vi "Begin.vi"(8 "error in":errorcluster) -> (0 "error out":errorcluster)   [LabVIEW 2016]
doc: "Called before other user functions, this VI can be used to open I/O refnums, load in file data, and do general program initialization. Notice that the <B>error out</B> terminal is simply used for data flow. Wiring it to other structures or subVIs ensures that this VI runs first."
uses:
  <vilib>/Rock Robotics/WPI/DriverStation/WPI_DriverStationRobotMode2.ctl
  <vilib>/Rock Robotics/WPI/Joystick/WPI_JoystickDeviceEnum.ctl
  <vilib>/Rock Robotics/SystemInterfaces/DIO/FPGA_DIOChannel.ctl
  <vilib>/Rock Robotics/WPI/Solenoid/WPI_SolenoidChannel.ctl
  <vilib>/Rock Robotics/SystemInterfaces/spilib/spi_bus.ctl
  <vilib>/Rock Robotics/WPI/SafetyOutput/WPI_SafetyOutputConfigMenu.ctl
  <vilib>/Rock Robotics/WPI/Encoder/WPI_EncoderType.ctl
  <vilib>/Rock Robotics/SystemInterfaces/DIO/FPGA_DIOPWMChannel.ctl
  <vilib>/Rock Robotics/SystemInterfaces/AI/FPGA_AIGyroChannel.ctl
  Robot Global Data.vi
  <vilib>/Rock Robotics/Network Tables/NT Write String Array.vi
  <vilib>/Rock Robotics/WPI/Counter/WPI_CounterDigitalInputToDigitalSource.vi
  <vilib>/Rock Robotics/WPI/Solenoid/WPI_SolenoidOpenDouble.vi
  <vilib>/Rock Robotics/WPI/MotorControl/WPI_MotorControlOpen SPARK.vi
  <vilib>/Rock Robotics/WPI/Gyro/WPI_GyroAnalogOpen.vi
  <vilib>/Rock Robotics/Network Tables/NT Read Number.vi
  <vilib>/Rock Robotics/WPI/Utilities/WPI_GetSetVariantRefNum.vi
  <vilib>/Rock Robotics/WPI/Solenoid/WPI_SolenoidOpenSingle.vi
  NavX/navX Library v2/navX Library v2.lvlib
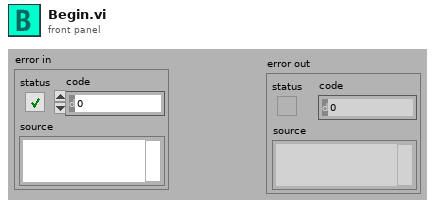
[diagram p1: front panel]
types:
  T1 = typedef "FPGA_AIGyroChannel.ctl" = enum8{"AI 0", "AI 1", "Invalid"}
  T2 = typedef "FPGA_DIOPWMChannel.ctl" = enum8{"PWM 0", "PWM 1", "PWM 2", "PWM 3", "PWM 4", "PWM 5", "PWM 6", "PWM 7", "PWM 8", "PWM 9", "PWM MXP 0", "PWM MXP 1", "PWM MXP 2", "PWM MXP 3", "PWM MXP 4", "PWM MXP 5", "PWM MXP 6", "PWM MXP 7", "PWM MXP 8", "PWM MXP 9", "Invalid"}
  T3 = typedef "FPGA_DIOChannel.ctl" = enum8{"DIO 0", "DIO 1", "DIO 2", "DIO 3", "DIO 4", "DIO 5", "DIO 6", "DIO 7", "DIO 8", "DIO 9", "DIO MXP 0", "DIO MXP 1", "DIO MXP 2", "DIO MXP 3", "DIO MXP 4", "DIO MXP 5", "DIO MXP 6", "DIO MXP 7", "DIO MXP 8", "DIO MXP 9", "DIO MXP 10", "DIO MXP 11", "DIO MXP 12", "DIO MXP 13", "DIO MXP 14", "DIO MXP 15", "SPI Port CS1", "SPI Port CS2", "SPI Port CS3", "SPI Port MISO", "SPI Port MOSI", "Invalid"}
  T4 = typedef "WPI_EncoderType.ctl" = enum16{"1x", "2x", "4x"}
  T5 = typedef "WPI_SafetyOutputConfigMenu.ctl" = enum16{"Enable", "Disable"}
  T6 = typedef "WPI_SolenoidChannel.ctl" = enum8{"Solenoid 0", "Solenoid 1", "Solenoid 2", "Solenoid 3", "Solenoid 4", "Solenoid 5", "Solenoid 6", "Solenoid 7", "Invalid"}
  T7 = typedef "WPI_JoystickDeviceEnum.ctl" = enum16{"USB 0", "USB 1", "USB 2", "USB 3", "USB 4", "USB 5"}
  T8 = typedef "spi_bus.ctl" = enum16{"SPI On-Board, CS0", "SPI On-Board, CS1", "SPI On-Board, CS2", "SPI On-Board, CS3", "SPI MXP", "Invalid"}
  T9 = typedef "WPI_DriverStationRobotMode2.ctl" = enum16{"Autonomous Disabled", "Autonomous Enabled", "Teleop Disabled", "Teleop Enabled", "Disconnected", "Finish", "Test Disabled", "Test Enabled", "Emergency Stopped"}
  T10 = typedef "WPI_CameraDevRef.ctl" = cluster{"Camera Address":string, "CameraStatus":errorcluster}
  T11 = typedef "WPI_GyroDevRef.ctl" = cluster{"DevStatus":errorcluster, "Analog Channel":T12, "Offset":dbl, "Gain (VoltsPerDegree/Second)":dbl, "Gyro Type":enum16{"Analog", "XRS450"}, "Handle":i32, "SPI Bus":T8, "Device Found":bool, "Sample Rate":dbl, "Calibrate On Open":bool}
  T12 = typedef "FPGA_AIChannel.ctl" = enum8{"AI 0", "AI 1", "AI 2", "AI 3", "AI MXP 0", "AI MXP 1", "AI MXP 2", "AI MXP 3", "Invalid"}
  T13 = typedef "WPI_JoystickDevRef.ctl" = cluster{"Device":T7}
  T14 = typedef "WPI_SolenoidDevRef.ctl" = cluster{"DevStatus":errorcluster, "Pneumatics Control Module":u8, "Forward Solenoid Channel":T6, "Reverse Solenoid Channel":T6}
  T15 = typedef "WPI_MotorControlDeviceRef.ctl" = cluster{"DeviceStatus":errorcluster, "Type":T16, "PWM":cluster{"PWM Channel":T2, "DeadBand":T17}, "CAN":cluster{"Device Number":u8, "SetOutput VI Ref":variant, "GetOutput VI Ref":variant, "Enable VI Ref":variant, "Disable VI Ref":variant, "Data":variant}, "Invert":bool}
  T16 = typedef "WPI_MotorControlType.ctl" = enum16{"PWM", "CAN"}
  T17 = typedef "WPI_PWMDeadband.ctl" = cluster{"Name":string, "maxPositivePwm":i32, "minPositivePwm":i32, "centerPwm":i32, "maxNegativePwm":i32, "minNegativePwm":i32, "angularRange":u16}
  T18 = typedef "WPI_DigitalInputDevRef.ctl" = cluster{"DevStatus":errorcluster, "DIO Channel":T3}
  T19 = typedef "FPGA_CounterEncoderSourceConvertionLVSourceType.ctl" = cluster{"DevStatus":errorcluster, "AnalogTriggerMode?":bool, "DigitalMode":cluster{"DIO Channel":T20}, "AnalogTriggerMode":cluster{"AnalogTriggerIndex":T21, "OutputType":T22}}
  T20 = typedef "FPGA_DIODigitalSourceChannel.ctl" = enum8{"DIO 0", "DIO 1", "DIO 2", "DIO 3", "DIO 4", "DIO 5", "DIO 6", "DIO 7", "DIO 8", "DIO 9", "DIO MXP 0", "DIO MXP 1", "DIO MXP 2", "DIO MXP 3", "DIO MXP 4", "DIO MXP 5", "DIO MXP 6", "DIO MXP 7", "DIO MXP 8", "DIO MXP 9", "DIO MXP 10", "DIO MXP 11", "DIO MXP 12", "DIO MXP 13", "DIO MXP 14", "DIO MXP 15", "Disabled"}
  T21 = typedef "FPGA_AnalogTriggerIndex.ctl" = enum8{"Trig 0", "Trig 1", "Trig 2", "Trig 3", "Trig 4", "Trig 5", "Trig 6", "Trig 7", "Invalid"}
  T22 = typedef "FPGA_AnalogTriggerOutType.ctl" = enum16{"InWindow", "TriggerState", "Rising", "Falling"}
  T23 = typedef "WPI_EncoderDevRef.ctl" = cluster{"DevStatus":errorcluster, "EncoderIndex":T24, "CounterIndex":T25, "DistancePerCount":dbl, "Decoding Type":T4}
  T24 = typedef "FPGA_EncoderIdx.ctl" = enum8{"Enc 0", "Enc 1", "Enc 2", "Enc 3", "Enc 4", "Enc 5", "Enc 6", "Enc 7", "Invalid"}
  T25 = typedef "FPGA_CounterCtrSystemIndex.ctl" = enum8{"Ctr 0", "Ctr 1", "Ctr 2", "Ctr 3", "Ctr 4", "Ctr 5", "Ctr 6", "Ctr 7", "Invalid"}
  T26 = typedef "navX Library v2.lvlib/Z900_navX_DeviceTypeDef.ctl" = cluster{"Interface":cluster{"Protocol":T27, "Update Rate (4Hz-60Hz)":u8, "navX Open TypeDef":variant}, "Notify Packet":refnum<notifier>, "Loop VI Refnum":refnum<vi>, "Ready to Close Occurrence Refnum":refnum<k4>}
  T27 = typedef "navX Library v2.lvlib/Z900_navX_ProtocolTypeDef.ctl" = enum16{"SERIAL", "I2C", "SPI"}
  T28 = cluster{"Yaw":dbl, "Roll":dbl, "Pitch":dbl, "Heading":dbl, "Fused Heading":dbl}
  T29 = typedef "WPI_CompressorDevRef.ctl" = cluster{"DevStatus":errorcluster, "Pneumatics Control Module":u8}
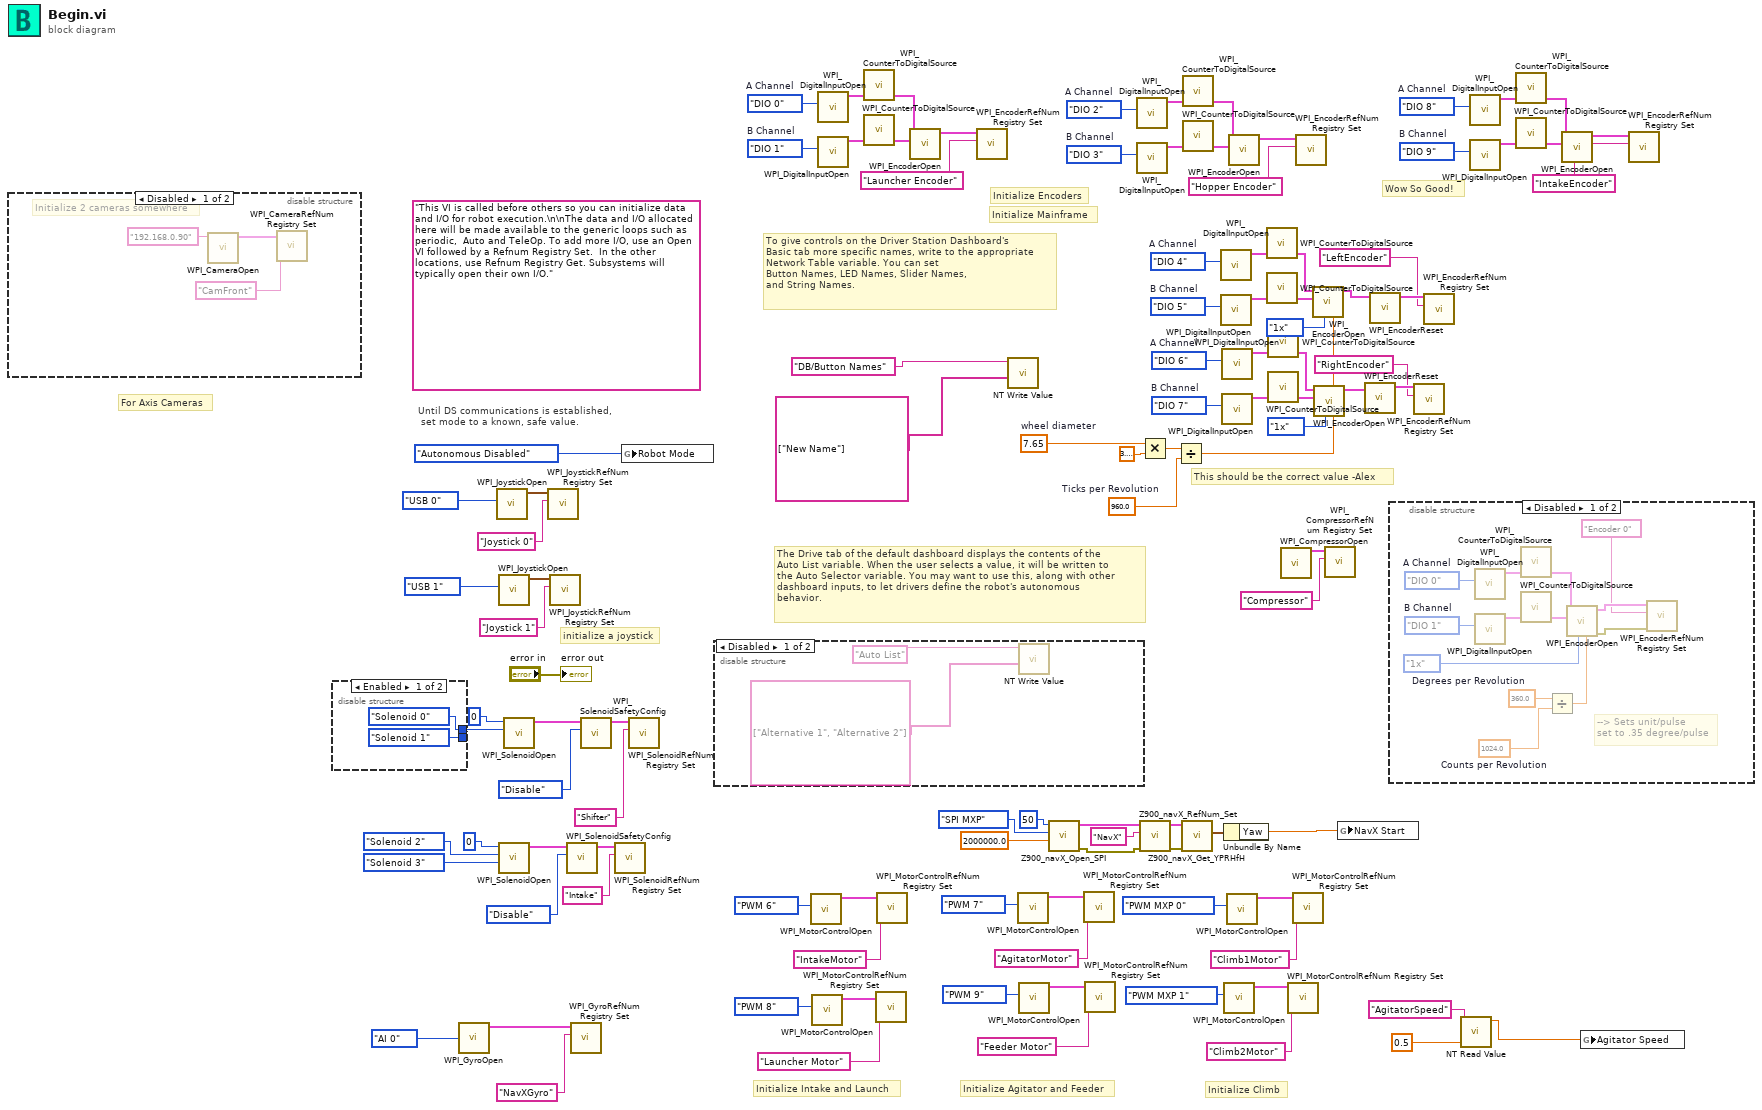
[diagram p0: block diagram]
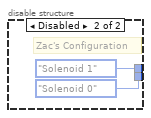
[diagram p4: hidden frame]
diagram:
  w25 = FPGA_DIOChannel."DIO 9"  # B Channel
  w26 = FPGA_DIOChannel."DIO 8"  # A Channel
  w41 = FPGA_DIOChannel."DIO 3"  # B Channel
  w42 = FPGA_DIOChannel."DIO 2"  # A Channel
  w33 = FPGA_DIOChannel."DIO 1"  # B Channel
  w34 = FPGA_DIOChannel."DIO 0"  # A Channel
  w52 = 960.0  # Ticks per Revolution
  w50 = 7.65  # wheel diameter
  w70 = FPGA_DIOChannel."DIO 5"  # B Channel
  w73 = FPGA_DIOChannel."DIO 4"  # A Channel
  w94 = FPGA_DIOChannel."DIO 7"  # B Channel
  w97 = FPGA_DIOChannel."DIO 6"  # A Channel
  (unwired) "This VI is called before others so you can initialize data and I/O for robot execution.\n\nThe data and I/O allocated here will be made available to the generic loops such as periodic,  Auto and TeleOp. To add more I/O, use an Open VI followed by a Refnum Registry Set.  In the other locations, use Refnum Registry Get. Subsystems will typically open their own I/O."
  # "Initialize Climb"
  # "Initialize Agitator and Feeder"
  # "Initialize Intake and Launch"
  # "For Axis Cameras"
  # "Wow So Good!"
  # "Initialize Mainframe"
  # "Initialize Encoders"
  # "This should be the correct value -Alex"
  # "The Drive tab of the default dashboard displays the contents of the\nAuto List variable. When the user selects a value, it will be written to\nthe Auto Selector variable. You may want to use this, along with other\ndashboard inputs, to let drivers define the robot's autonomous\nbehavior."
  # "To give controls on the Driver Station Dashboard's\nBasic tab more specific names, write to the appropriate\nNetwork Table variable. You can set\nButton Names, LED Names, Slider Names,\nand String Names."
  # "initialize a joystick"
  # "Until DS communications is established,\n set mode to a known, safe value."
  n1 = disable-structure shown="Disabled" {
    frame Disabled {
      # "Initialize 2 cameras somewhere"
      n2 = call <vilib>:"WPI_CameraOpen.vi"("Camera Address"="192.168.0.90") -> ("CameraDevRef"=w111:T10)  [unwired: 9 in, 1 out]
      n3 = call <vilib>:"WPI_CameraRefNum Registry Set.vi"("refnum name"="CamFront", "CameraDevRef"=w111) -> ()  [unwired: 8 in, 2 out]
    }
    frame Enabled {
    }
  }
  n4 = disable-structure shown="Enabled" {
    disable-tunnel: [WPI_SolenoidChannel."Solenoid 0" ("Solenoid Channel") WPI_SolenoidChannel."Solenoid 1" ("Solenoid Channel")] -> w79
    disable-tunnel: [WPI_SolenoidChannel."Solenoid 1" ("Reverse Solenoid Channel") WPI_SolenoidChannel."Solenoid 0" ("Reverse Solenoid Channel")] -> _
    frame Enabled {
    }
    frame Disabled {
      # "Zac's Configuration"
    }
  }
  n5 = call-poly <vilib>:"WPI_GyroOpen.vi"("Analog Channel"=FPGA_AIGyroChannel."AI 0") -> ("GyroDevRef"=w5:T11)  [unwired: 8 in, 2 out]
  n6 = call <vilib>:"WPI_JoystickOpen.vi"("JoystickDevice"=WPI_JoystickDeviceEnum."USB 0") -> ("JoystickDevRef"=w106:T13)  [unwired: 10 in]
  n7 = call <vilib>:"WPI_JoystickOpen.vi"("JoystickDevice"=WPI_JoystickDeviceEnum."USB 1") -> ("JoystickDevRef"=w68:T13)  [unwired: 10 in]
  n8 = call-poly <vilib>:"WPI_SolenoidOpen.vi"("Reverse Solenoid Channel"=WPI_SolenoidChannel."Solenoid 3", "Forward Solenoid Channel"=WPI_SolenoidChannel."Solenoid 2" ("Solenoid Channel"), "Pneumatics Control Module (0)"=u8 0) -> ("SolenoidDevRef"=w92:T14)  [unwired: 7 in, 1 out]
  n9 = call-poly <vilib>:"WPI_SolenoidOpen.vi"("Solenoid Channel"=w79, "Pneumatics Control Module (0)"=u8 0) -> ("SolenoidDevRef"=w62:T14)  [unwired: 8 in, 1 out]
  n10 = call <vilib>:"WPI_JoystickRefNum Registry Set.vi"("refnum name"="Joystick 0", "JoystickDevRef"=w106) -> ()  [unwired: 8 in, 2 out]
  n11 = call <vilib>:"WPI_JoystickRefNum Registry Set.vi"("refnum name"="Joystick 1", "JoystickDevRef"=w68) -> ()  [unwired: 8 in, 2 out]
  n12 = call <vilib>:"WPI_SolenoidSafetyConfig.vi"("mode"=WPI_SafetyOutputConfigMenu."Disable", "SolenoidDevRef"=w92) -> ("SolenoidDevRef"=w59:T14)  [unwired: 8 in, 1 out]
  n13 = call <vilib>:"WPI_GyroRefNum Registry Set.vi"("refnum name"="NavXGyro", "GyroDevRef"=w5) -> ()  [unwired: 8 in, 2 out]
  n14 = call <vilib>:"WPI_SolenoidSafetyConfig.vi"("mode"=WPI_SafetyOutputConfigMenu."Disable", "SolenoidDevRef"=w62) -> ("SolenoidDevRef"=w61:T14)  [unwired: 8 in, 1 out]
  n15 = call <vilib>:"WPI_SolenoidRefNum Registry Set.vi"("refnum name"="Intake", "SolenoidDevRef"=w59) -> ()  [unwired: 8 in, 2 out]
  n16 = global write "Robot Global Data.vi" "Robot Mode"(WPI_DriverStationRobotMode2."Autonomous Disabled" ("Robot Mode")) -> ()
  n17 = call <vilib>:"WPI_SolenoidRefNum Registry Set.vi"("refnum name"="Shifter", "SolenoidDevRef"=w61) -> ()  [unwired: 8 in, 2 out]
  n18 = disable-structure shown="Disabled" {
    frame Disabled {
      n19 = call-poly <vilib>:"NT Write Value.vi"("String Array"=string[] ["Alternative 1", "Alternative 2"], "Name"="Auto List") -> ()  [unwired: 9 in, 1 out]
    }
    frame Enabled {
    }
  }
  n20 = call-poly <vilib>:"WPI_MotorControlOpen.vi"("PWM Channel"=FPGA_DIOPWMChannel."PWM 6") -> ("MotorControlDeviceRef"=w11:T15)  [unwired: 9 in, 1 out]
  n21 = call-poly <vilib>:"WPI_MotorControlOpen.vi"("PWM Channel"=FPGA_DIOPWMChannel."PWM 8") -> ("MotorControlDeviceRef"=w8:T15)  [unwired: 9 in, 1 out]
  n22 = call <vilib>:"WPI_DigitalInputOpen.vi"("DIO Channel"=w34) -> ("DigitalInputDevRef"=w37:T18)  [unwired: 1 in, 9 out]
  n23 = call <vilib>:"WPI_DigitalInputOpen.vi"("DIO Channel"=w33) -> ("DigitalInputDevRef"=w36:T18)  [unwired: 1 in, 9 out]
  n24 = call-poly <vilib>:"WPI_CounterToDigitalSource.vi"("DigitalInputDevRef"=w37) -> ("Digital Source"=w38:T19)  [unwired: 6 out]
  n25 = call-poly <vilib>:"WPI_CounterToDigitalSource.vi"("DigitalInputDevRef"=w36) -> ("Digital Source"=w35:T19)  [unwired: 6 out]
  n26 = call <vilib>:"WPI_MotorControlRefNum Registry Set.vi"("refnum name"="Launcher Motor", "MotorControlDevRef"=w8) -> ()  [unwired: 8 in, 2 out]
  n27 = call <vilib>:"WPI_MotorControlRefNum Registry Set.vi"("refnum name"="IntakeMotor", "MotorControlDevRef"=w11) -> ()  [unwired: 8 in, 2 out]
  n28 = call <vilib>:"WPI_EncoderOpen.vi"("BSource"=w35, "ASource"=w38) -> ("EncoderDevRef"=w39:T23)  [unwired: 6 in, 3 out]
  n29 = call <vilib>:"WPI_EncoderRefNum Registry Set.vi"("refnum name"="Launcher Encoder", "EncoderDevRef"=w39) -> ()  [unwired: 8 in, 2 out]
  n30 = call-poly <vilib>:"NT Write Value.vi"("String Array"=string[] ["New Name"], "Name"="DB/Button Names") -> ()  [unwired: 9 in, 1 out]
  n31 = call-poly <vilib>:"WPI_MotorControlOpen.vi"("PWM Channel"=FPGA_DIOPWMChannel."PWM 7") -> ("MotorControlDeviceRef"=w14:T15)  [unwired: 9 in, 1 out]
  n32 = call-poly <vilib>:"WPI_MotorControlOpen.vi"("PWM Channel"=FPGA_DIOPWMChannel."PWM 9") -> ("MotorControlDeviceRef"=w16:T15)  [unwired: 9 in, 1 out]
  n33 = call "Z900_navX_Open_SPI.vi"("Clock Rate (Hz)"=2000000.0, "SPI Bus"=spi_bus."SPI MXP", "Update Rate (4Hz-60Hz)"=u8 50) -> ("error out"=w57:errorcluster, "navX Device"=w85:T26)  [unwired: 7 in]
  n34 = call <vilib>:"WPI_MotorControlRefNum Registry Set.vi"("refnum name"="AgitatorMotor", "MotorControlDevRef"=w14) -> ()  [unwired: 8 in, 2 out]
  n35 = call <vilib>:"WPI_MotorControlRefNum Registry Set.vi"("refnum name"="Feeder Motor", "MotorControlDevRef"=w16) -> ()  [unwired: 8 in, 2 out]
  n36 = call <vilib>:"WPI_DigitalInputOpen.vi"("DIO Channel"=w42) -> ("DigitalInputDevRef"=w45:T18)  [unwired: 1 in, 9 out]
  n37 = call <vilib>:"WPI_DigitalInputOpen.vi"("DIO Channel"=w41) -> ("DigitalInputDevRef"=w44:T18)  [unwired: 1 in, 9 out]
  n38 = Multiply(x=w50, y=3.141592653589793) -> (x*y=w53:dbl)
  n39 = call "Z900_navX_RefNum_Set.vi"("error in (no error)"=w57, "refnum name"="NavX", "navX Device"=w85) -> ("error out"=w56:errorcluster, "navX Device"=w86:T26)  [unwired: 7 in]
  n40 = Divide(x=w53, y=w52) -> (x/y=w49:dbl)
  n41 = call "Z900_navX_Get_YPRHfH.vi"("error in (no error)"=w56, "navX Device"=w86) -> ("YRPHfH"=w87:T28)  [unwired: 6 in, 3 out]
  n42 = call-poly <vilib>:"WPI_CounterToDigitalSource.vi"("DigitalInputDevRef"=w45) -> ("Digital Source"=w46:T19)  [unwired: 6 out]
  n43 = call-poly <vilib>:"WPI_CounterToDigitalSource.vi"("DigitalInputDevRef"=w44) -> ("Digital Source"=w43:T19)  [unwired: 6 out]
  n44 = call <vilib>:"WPI_DigitalInputOpen.vi"("DIO Channel"=w73) -> ("DigitalInputDevRef"=w74:T18)  [unwired: 1 in, 9 out]
  n45 = call <vilib>:"WPI_DigitalInputOpen.vi"("DIO Channel"=w70) -> ("DigitalInputDevRef"=w71:T18)  [unwired: 1 in, 9 out]
  n46 = call <vilib>:"WPI_DigitalInputOpen.vi"("DIO Channel"=w97) -> ("DigitalInputDevRef"=w98:T18)  [unwired: 1 in, 9 out]
  n47 = call <vilib>:"WPI_DigitalInputOpen.vi"("DIO Channel"=w94) -> ("DigitalInputDevRef"=w95:T18)  [unwired: 1 in, 9 out]
  n48 = Unbundle By Name(w87) -> ("Yaw"=w88:dbl)
  n49 = call-poly <vilib>:"WPI_MotorControlOpen.vi"("PWM Channel"=FPGA_DIOPWMChannel."PWM MXP 1") -> ("MotorControlDeviceRef"=w20:T15)  [unwired: 9 in, 1 out]
  n50 = call-poly <vilib>:"WPI_MotorControlOpen.vi"("PWM Channel"=FPGA_DIOPWMChannel."PWM MXP 0") -> ("MotorControlDeviceRef"=w22:T15)  [unwired: 9 in, 1 out]
  n51 = call <vilib>:"WPI_EncoderOpen.vi"("BSource"=w43, "ASource"=w46) -> ("EncoderDevRef"=w47:T23)  [unwired: 6 in, 3 out]
  n52 = call-poly <vilib>:"WPI_CounterToDigitalSource.vi"("DigitalInputDevRef"=w74) -> ("Digital Source"=w75:T19)  [unwired: 6 out]
  n53 = call-poly <vilib>:"WPI_CounterToDigitalSource.vi"("DigitalInputDevRef"=w71) -> ("Digital Source"=w72:T19)  [unwired: 6 out]
  n54 = call-poly <vilib>:"WPI_CounterToDigitalSource.vi"("DigitalInputDevRef"=w98) -> ("Digital Source"=w99:T19)  [unwired: 6 out]
  n55 = call-poly <vilib>:"WPI_CounterToDigitalSource.vi"("DigitalInputDevRef"=w95) -> ("Digital Source"=w96:T19)  [unwired: 6 out]
  n56 = call <vilib>:"WPI_CompressorOpen.vi"() -> ("CompressorDevRef"=w64:T29)  [unwired: 14 in, 1 out]
  n57 = call <vilib>:"WPI_MotorControlRefNum Registry Set.vi"("refnum name"="Climb2Motor", "MotorControlDevRef"=w20) -> ()  [unwired: 8 in, 2 out]
  n58 = call <vilib>:"WPI_MotorControlRefNum Registry Set.vi"("refnum name"="Climb1Motor", "MotorControlDevRef"=w22) -> ()  [unwired: 8 in, 2 out]
  n59 = call <vilib>:"WPI_EncoderRefNum Registry Set.vi"("refnum name"="Hopper Encoder", "EncoderDevRef"=w47) -> ()  [unwired: 8 in, 2 out]
  n60 = call <vilib>:"WPI_EncoderOpen.vi"("DistancePerCount"=w49, "Decoding Type"=WPI_EncoderType."1x", "BSource"=w72, "ASource"=w75) -> ("EncoderDevRef"=w76:T23)  [unwired: 4 in, 3 out]
  n61 = call <vilib>:"WPI_EncoderOpen.vi"("DistancePerCount"=w49, "Decoding Type"=WPI_EncoderType."1x", "BSource"=w96, "ASource"=w99) -> ("EncoderDevRef"=w100:T23)  [unwired: 4 in, 3 out]
  n62 = call <vilib>:"WPI_CompressorRefNum Registry Set.vi"("refnum name"="Compressor", "CompressorDevRef"=w64) -> ()  [unwired: 8 in, 2 out]
  n63 = global write "Robot Global Data.vi" "NavX Start"(w88) -> ()
  n64 = call <vilib>:"WPI_EncoderReset.vi"("EncoderDevRef"=w100) -> ("EncoderDevRef"=w101:T23)  [unwired: 9 in, 1 out]
  n65 = call <vilib>:"WPI_EncoderReset.vi"("EncoderDevRef"=w76) -> ("EncoderDevRef"=w77:T23)  [unwired: 9 in, 1 out]
  n66 = disable-structure shown="Disabled" {
    frame Disabled {
      w118 = 360.0  # Degrees per Revolution
      w121 = 1024.0  # Counts per Revolution
      w130 = FPGA_DIOChannel."DIO 1"  # B Channel
      w129 = FPGA_DIOChannel."DIO 0"  # A Channel
      # "--> Sets unit/pulse\nset to .35 degree/pulse"
      n67 = call <vilib>:"WPI_DigitalInputOpen.vi"("DIO Channel"=w129) -> ("DigitalInputDevRef"=w126:T18)  [unwired: 1 in, 9 out]
      n68 = call <vilib>:"WPI_DigitalInputOpen.vi"("DIO Channel"=w130) -> ("DigitalInputDevRef"=w127:T18)  [unwired: 1 in, 9 out]
      n69 = call-poly <vilib>:"WPI_CounterToDigitalSource.vi"("DigitalInputDevRef"=w126) -> ("Digital Source"=w125:T19)  [unwired: 6 out]
      n70 = call-poly <vilib>:"WPI_CounterToDigitalSource.vi"("DigitalInputDevRef"=w127) -> ("Digital Source"=w128:T19)  [unwired: 6 out]
      n71 = Divide(x=w118, y=w121) -> (x/y=w120:dbl)
      n72 = call <vilib>:"WPI_EncoderOpen.vi"("DistancePerCount"=w120, "Decoding Type"=WPI_EncoderType."1x", "BSource"=w128, "ASource"=w125) -> ("error out"=w123:errorcluster, "EncoderDevRef"=w124:T23)  [unwired: 4 in, 2 out]
      n73 = call <vilib>:"WPI_EncoderRefNum Registry Set.vi"("error in (no error)"=w123, "refnum name"="Encoder 0", "EncoderDevRef"=w124) -> ()  [unwired: 7 in, 2 out]
    }
    frame Enabled {
    }
  }
  n74 = call <vilib>:"WPI_EncoderRefNum Registry Set.vi"("refnum name"="RightEncoder", "EncoderDevRef"=w101) -> ()  [unwired: 8 in, 2 out]
  n75 = call <vilib>:"WPI_EncoderRefNum Registry Set.vi"("refnum name"="LeftEncoder", "EncoderDevRef"=w77) -> ()  [unwired: 8 in, 2 out]
  n76 = call-poly <vilib>:"NT Read Value.vi"("Default Value"=0.5, "Name"="AgitatorSpeed") -> ("Numeric"=w1:dbl)  [unwired: 8 in, 1 out]
  n77 = call <vilib>:"WPI_DigitalInputOpen.vi"("DIO Channel"=w26) -> ("DigitalInputDevRef"=w29:T18)  [unwired: 1 in, 9 out]
  n78 = call <vilib>:"WPI_DigitalInputOpen.vi"("DIO Channel"=w25) -> ("DigitalInputDevRef"=w28:T18)  [unwired: 1 in, 9 out]
  n79 = call-poly <vilib>:"WPI_CounterToDigitalSource.vi"("DigitalInputDevRef"=w29) -> ("Digital Source"=w30:T19)  [unwired: 6 out]
  n80 = call-poly <vilib>:"WPI_CounterToDigitalSource.vi"("DigitalInputDevRef"=w28) -> ("Digital Source"=w27:T19)  [unwired: 6 out]
  n81 = call <vilib>:"WPI_EncoderOpen.vi"("BSource"=w27, "ASource"=w30) -> ("EncoderDevRef"=w31:T23)  [unwired: 6 in, 3 out]
  n82 = global write "Robot Global Data.vi" "Agitator Speed"(w1) -> ()
  n83 = call <vilib>:"WPI_EncoderRefNum Registry Set.vi"("refnum name"="IntakeEncoder", "EncoderDevRef"=w31) -> ()  [unwired: 8 in, 2 out]
  "error out" <- "error in"
